vi "Get Board Number.vi"(8 "error in (no error)":errorcluster, 11 "Pulseblaster in":refnum<class "Slave_Pulseblaster.lvclass">) -> (0 "error out":errorcluster, 2 "Board Number":i32 max=256 step=1, 3 "Pulseblaster out":refnum<class "Slave_Pulseblaster.lvclass">)   [LabVIEW 2013, in "Slave_Pulseblaster.lvclass"]
uses:
  Slave_Pulseblaster.lvclass
  Slave_Pulseblaster.lvclass/Slave_Pulseblaster.ctl
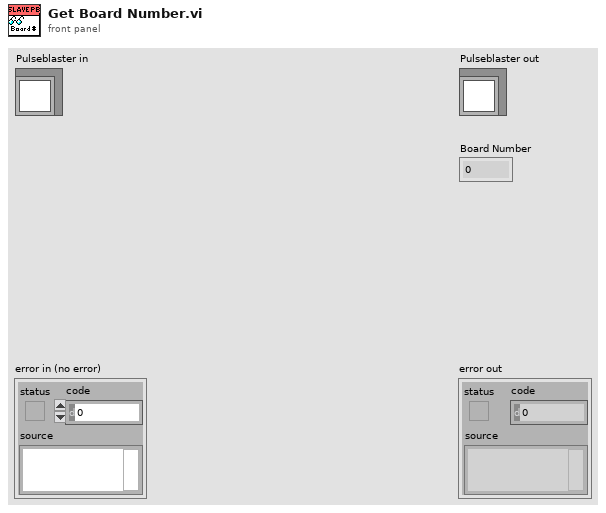
[diagram p1: front panel]
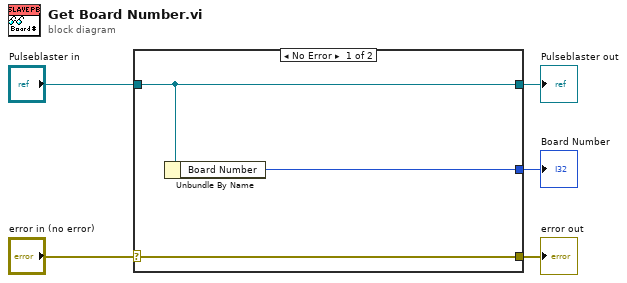
[diagram p0: block diagram]
diagram:
  n1 = case shown="No Error" "error in (no error)" {
    selector: "error in (no error)" -> [w8 w9]
    tunnel: [w8 w9] -> w4
    tunnel: [w7 w10] -> w2
    tunnel: "Pulseblaster in" -> [w7 w10]
    tunnel: [w6 _] -> w1
    frame No Error {
      n2 = Unbundle By Name(w7) -> ("Board Number"=w6:i32)
    }
    frame Error {
    }
  }
  "error out" <- w4
  "Pulseblaster out" <- w2
  "Board Number" <- w1
